vi "[RT] Cont Acq.vi"() -> ()   [LabVIEW 2015]
doc: "The continuous acquisition mode tells the FPGA to acquire points indefinitely until a stop command is issued or until an error is encountered (FIFO overflow, module underflow, and so on). \n\nIn this acquisition mode, explicitly call the appropriate rwfm_ConfigTiming VI and set the host application's data buffer to be many times larger than the read size. The examples use a 10X size by default. If the host application's data buffer fills, then the FPGA experiences a FIFO overflow causing the acquisition to stop."
uses:
  <vilib>/NI/cRIO Wfm/ChannelConfig.ctl
  <vilib>/FPGAPlugInAG/sbRIO-9607/niLvFpga_Open_sbRIO-9607.vi
  <vilib>/rvi/interface/common/dynamic/niFpgaDynamicAddResources.vi
  <vilib>/FPGAPlugInAG/Dynamic/niLvFpga_Reset_Dynamic.vi
  <vilib>/FPGAPlugInAG/Dynamic/niLvFpga_Run_Dynamic.vi
  <vilib>/FPGAPlugInAG/Dynamic/niLvFpga_Close_Dynamic.vi
  <vilib>/rvi/interface/nirviOpenFPGA/nirviOpenFPGA.xnode
  FPGA Bitfiles/WaveformLibraryI_FPGATarget2_[FPGA]SARAcqMain_U+qOsuK4w1s.lvbitx
  FPGA/[FPGA] SAR Acq Main.vi
  <vilib>/rvi/interface/nirviMethod/nirviMethod.xnode
  <vilib>/rvi/interface/nirviCloseFPGA/nirviCloseFPGA.xnode
  IFw_Addon/RT/WaveformTask.lvclass
  <vilib>/NI/cRIO Wfm/cRIO Wfm.lvlib
panel:
  in  "Sample Rate":u32=51200
  in  "stop":bool
  out "Waveform Graph":waveform(sgl)[](graph)
  in  "Channel Info":T1=[{"Channel Name"="Mod1/ai0", "Sensitivity mV_EU"=1000.0, "EU"="V", "dB Ref EU"=1.0}, {"Channel Name"="Mod1/ai1", "Sensitivity mV_EU"=1000.0, "EU"="V", "dB Ref EU"=1.0}, {"Channel Name"="Mod1/ai2", "Sensitivity mV_EU"=1000.0, "EU"="V", "dB Ref EU"=1.0}] caption="Channel Name      Scale [mV/EU]        EU           dB Ref [EU]" {"dB Ref EU" format="%#.2p"; "Sensitivity mV_EU" format="%.2f"}
  in  "Samps per Chan":i32=25600 caption="Samples per Channel"
  out "Buffer Backlog":dbl caption="RT Buffer Backlog [%]" format="%#.2g"
  # "Sampling Info"
  # "Channel Info"
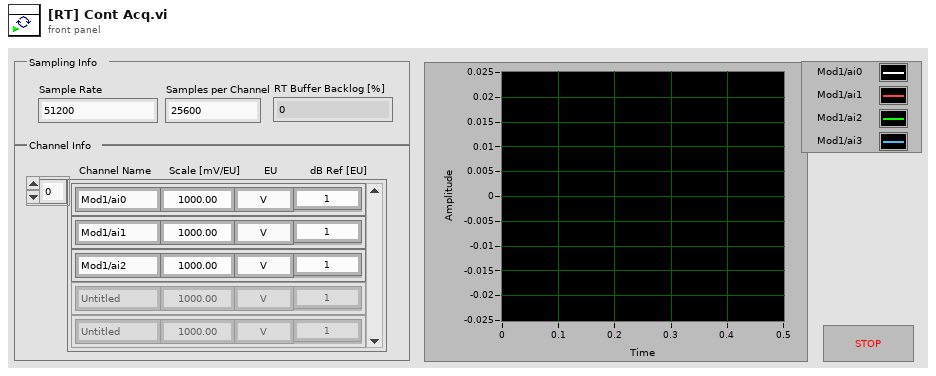
[diagram p1: front panel]
types:
  T1 = typedef "cRIO Wfm.lvlib/ChannelConfig.ctl" = cluster{"Channel Name":string, "Sensitivity mV_EU":dbl, "EU":string, "dB Ref EU":dbl}[]
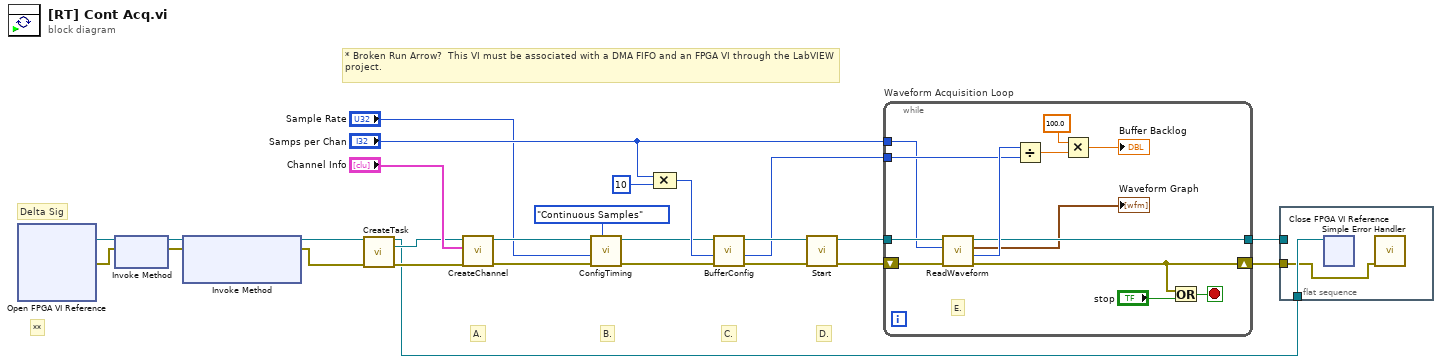
[diagram p0: block diagram]
diagram:
  # "Delta Sig"
  # "**"
  # "* Broken Run Arrow?  This VI must be associated with a DMA FIFO and an FPGA VI through the LabVIEW project."
  # "D."
  # "C."
  # "B."
  # "A."
  n1 = xnode "Open FPGA VI Reference"() -> ("FPGA VI Reference Out"=w9:refnum<k20>, "error out"=w8:errorcluster)  [unwired: 2 in]
  n2 = xnode "Invoke Method"("FPGA VI Reference In"=w9, "error in"=w8) -> ("FPGA VI Reference Out"=w11:refnum<k20>, "error out"=w10:errorcluster)
  n3 = xnode "Invoke Method"("FPGA VI Reference In"=w11, "error in"=w10) -> ("FPGA VI Reference Out"=w7:refnum<k20>, "error out"=w6:errorcluster)  [unwired: 1 in]
  n4 = call "CreateTask.vi"("FPGA Ref in"=w7, "error in"=w6) -> ("FPGA Ref out"=w1:refnum<k20>, "Task out"=w4:refnum<class "WaveformTask.lvclass">, "error out"=w5:errorcluster)  [unwired: 11 in]
  n5 = call "CreateChannel.vi"("error in"=w5, "Channel Info"="Channel Info", "task in"=w4) -> ("error out"=w14:errorcluster, "Task out"=w17:refnum<class "WaveformTask.lvclass">)  [unwired: 7 in]
  n6 = call "ConfigTiming.vi"("Sample Mode"=enum16{"Finite Samples", "Continuous Samples"}."Continuous Samples", "error in (no error)"=w14, "Sample Rate"="Sample Rate", "Task in"=w17) -> ("error out"=w15:errorcluster, "Task out"=w16:refnum<class "WaveformTask.lvclass">)  [unwired: 5 in, 1 out]
  n7 = Compound Arithmetic op=MULTIPLY("Samps per Chan", 10 ("value")) -> (w20:i32)
  n8 = call "BufferConfig.vi"("error in (no error)"=w15, "Buffer Size [Samps per Chan]"=w20, "WaveformTask in"=w16) -> ("error out"=w21:errorcluster, "Buffer Size [Total Samples]"=w19:u32, "WaveformTask out"=w22:refnum<class "WaveformTask.lvclass">)  [unwired: 6 in]
  n9 = call "Start.vi"("error in (no error)"=w21, "WaveformTask in"=w22) -> ("error out"=w25:errorcluster, "WaveformTask out"=w26:refnum<class "WaveformTask.lvclass">)  [unwired: 8 in]
  n10 = while "Waveform Acquisition Loop" {
    tunnel: w26 -> [w33]
    tunnel: [w29] -> w2
    tunnel: w19 -> [w37]
    tunnel: "Samps per Chan" -> [w30]
    shift-right: [w28] -> w24
    shift-left: w25 -> [w39]
    stop <- w32 stop-if-true
    # "E."
    n11 = call "ReadWaveform.vi"("error in"=w39, "Samps Read per Chan"=w30, "Task in"=w33) -> ("error out"=w28:errorcluster, "Samples Remaining"=w38:u32, "Waveforms"=→"Waveform Graph":waveform(sgl)[], "Task out"=w29:refnum<class "WaveformTask.lvclass">)  [unwired: 5 in]
    n12 = Divide(x=w38, y=w37) -> (x/y=w36:dbl)
    n13 = Multiply(x=100.0, y=w36) -> (x*y=→"Buffer Backlog":dbl)
    n14 = Or(x=w28, y="stop") -> (x .or. y?=w32:bool)
  }
  n15 = flat-sequence {
    tunnel: w24 -> [w40]
    tunnel: w2 -> [_]
    tunnel: w1 -> [w41]
    frame #0 {
      n16 = xnode "Close FPGA VI Reference"("FPGA VI Reference In"=w41) -> ()  [unwired: 1 in, 1 out]
      n17 = call <vilib>:"Simple Error Handler.vi"("error in (no error)"=w40) -> ()  [unwired: 1 in, 8 out]
    }
  }
